vi "Convert Callback To Dbl Click.vi"(6 "Return Meet Filter Selection (T)":bool=TRUE, 8 "error in":errorcluster, 10 "Data":variant, 11 "TreeAliasBrowser Ref":T2) -> (0 "error out":errorcluster, 2 "Valid?":bool, 3 "Selected Node":T1)   [LabVIEW 2020, in "NI_VS UI Tree Alias Browser.lvlib"]
uses:
  <vilib>/NI VeriStand/UI Controls/Tree and Alias Browser/NI_VS UI Tree Alias Browser.lvlib
  <vilib>/NI VeriStand/UI Controls/Tree and Alias Browser/Tree Alias Browser Ref.ctl
  NationalInstruments.VeriStand.SystemStorageUI
  <vilib>/NI VeriStand/UI Controls/Tree and Alias Browser/Node Ref.ctl
  NationalInstruments.VeriStand.SystemStorage
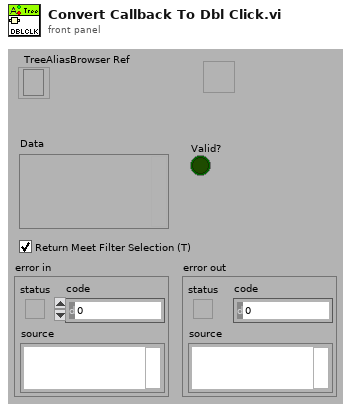
[diagram p1: front panel]
types:
  T1 = typedef "NI_VS UI Tree Alias Browser.lvlib/Node Ref.ctl" = refnum<k24>
  T2 = typedef "NI_VS UI Tree Alias Browser.lvlib/Tree Alias Browser Ref.ctl" = refnum<k24>
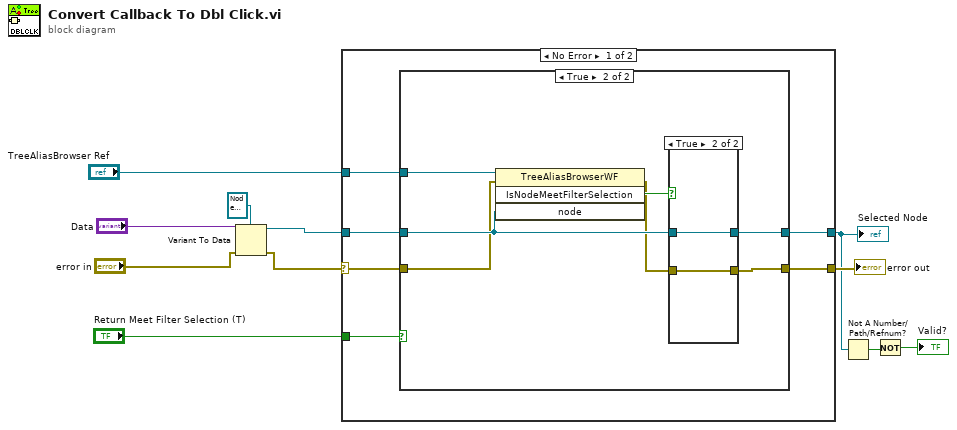
[diagram p0: block diagram]
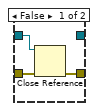
[diagram p3: hidden frame]
diagram:
  n1 = Variant To Data(error in="error in", type=T1 refnum ("Selected Node"), Variant="Data") -> (data=w8:T1, error out=w9:errorcluster)
  n2 = case shown="No Error" w9 {
    selector: w9 -> [w14 w32]
    tunnel: "TreeAliasBrowser Ref" -> [w17 _]
    tunnel: w8 -> [w15 _]
    tunnel: "Return Meet Filter Selection (T)" -> [w16 _]
    tunnel: [w13 w32] -> w6
    tunnel: [w12 _] -> w2
    frame No Error {
      n3 = case shown="True" w16 {
        tunnel: w17 -> [_ w26]
        tunnel: w15 -> [w18 w25]
        tunnel: w14 -> [w19 w24]
        tunnel: [w19 w23] -> w13
        tunnel: [w18 w20] -> w12
        frame False {
        }
        frame True {
          n4 = invoke class="TreeAliasBrowserWF" method="IsNodeMeetFilterSelection"(reference=w26, error in=w24, "node"=w25) -> (error out=w21:errorcluster, "IsNodeMeetFilterSelection"=w22:bool)  [unwired: 1 in, 2 out]
          n5 = case shown="True" w22 {
            tunnel: w25 -> [w29 w30]
            tunnel: w21 -> [w28 w31]
            tunnel: [w27 w31] -> w23
            tunnel: [_ w30] -> w20
            frame False {
              n6 = Close Reference(reference=w29, error in (no error)=w28) -> (error out=w27:errorcluster)
            }
            frame True {
            }
          }
        }
      }
    }
    frame Error {
    }
  }
  "error out" <- w6
  "Selected Node" <- w2
  n7 = Not A Number/Path/Refnum?(number/path/refnum=w2) -> (NaN/Path/Refnum?=w5:bool)
  n8 = Not(x=w5) -> (.not. x?=→"Valid?":bool)
